vi "RSZVB Set Signal Power Mode.vi"(7 "Mode (Fixed)":i32(ring) items=["Fixed", "Fundamental"], 8 "error in (no error)":errorcluster {"code" format="%.0x"}, 9 "Signal (RF)":i32(ring) items=["RF"=0, "IF"=2, "LO 1"=3, "LO 2"=4, "Aux LO"=5], 10 "Channel (1)":i32=1, 11 "VISA resource name":refnum<visa-resource-name>) -> (0 "error out":errorcluster {"code" format="%.0x"}, 3 "VISA resource name out":refnum<visa-resource-name>)   [LabVIEW 2011]
doc: "This VI sets the RF, LO 1, LO 2, Aux LO, or the IF signal ports to fixed power or to the channel base power.\n\nRemote-control command(s):\nSOURce<Ch>:FREQuency<Pt>:CONVersion:MIXer:PMODe RF | LO | LO1 | LO2 | AUXLo | IF, FIXed | FUNDamental"
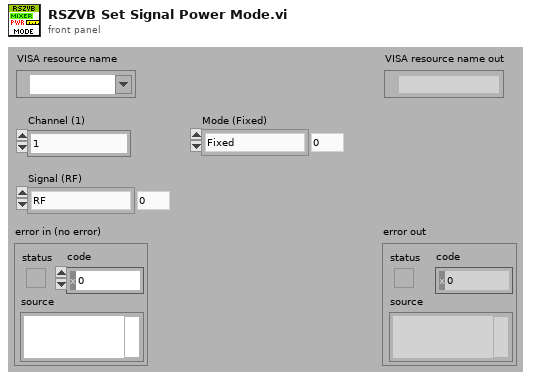
[diagram p1: front panel]
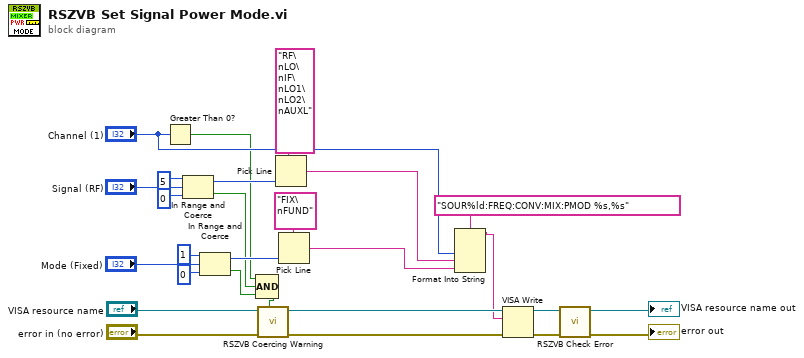
[diagram p0: block diagram]
diagram:
  n1 = Greater Than 0?(x="Channel (1)") -> (x > 0?=w2:bool)
  n2 = In Range and Coerce(upper limit=5, x="Signal (RF)", lower limit=0) -> (coerced(x)=w16:i32, In Range?=w1:bool)
  n3 = In Range and Coerce(upper limit=1, x="Mode (Fixed)", lower limit=0) -> (coerced(x)=w4:i32, In Range?=w18:bool)
  n4 = Compound Arithmetic op=AND(w2, w1, w18) -> (w23:bool)
  n5 = call "RSZVB Coercing Warning.vi"("In Range?"=w23, "error in (no error)"="error in (no error)", "VISA session"="VISA resource name") -> ("error out"=w26:errorcluster, "dup VISA session"=w27:refnum<visa-resource-name>)  [unwired: 7 in]
  n6 = Pick Line(multi-line string="RF\nLO\nIF\nLO1\nLO2\nAUXL", line index=w16) -> (output string=w13:string)  [unwired: 1 in]
  n7 = Pick Line(multi-line string="FIX\nFUND", line index=w4) -> (output string=w3:string)  [unwired: 1 in]
  n8 = Format Into String(format string="SOUR%ld:FREQ:CONV:MIX:PMOD %s,%s", "Channel (1)", w13, w3) -> (resulting string=w19:string)  [unwired: 2 in, 1 out]
  n9 = VISA Write(VISA resource name=w27, write buffer=w19, error in (no error)=w26) -> (VISA resource name out=w24:refnum<visa-resource-name>, error out=w25:errorcluster)  [unwired: 1 out]
  n10 = call "RSZVB Check Error.vi"("error in (no error)"=w25, "VISA session"=w24) -> ("error out"=→"error out":errorcluster, "dup VISA session"=→"VISA resource name out":refnum<visa-resource-name>)  [unwired: 8 in]
